vi "Build-raw-path.vi"(8 "error in (no error)":errorcluster, 11 "Reference in":T3) -> (0 "error out":errorcluster, 2 "Path":T1[](array[typedef]), 3 "Reference out":T3)   [LabVIEW 2013, in "HardwareCharacterization.lvlib" / "HC-ScanParser.lvclass"]
uses:
  HC-ScanParser.lvclass
  Object-reference.ctl
  Point-buffer.ctl
  SM1000-XML/Element-XML/Elements.ctl
  Path-buffer.ctl
  Property-buffer.ctl
  Units.ctl
  Speed.ctl
  HC-ScanParser.lvclass/HC-ScanParser.ctl
  SM1000-XML/Element-XML/Element-XML.lvclass
  Read Field properties.vi
  Read Laser properties.vi
  Read Elements.vi
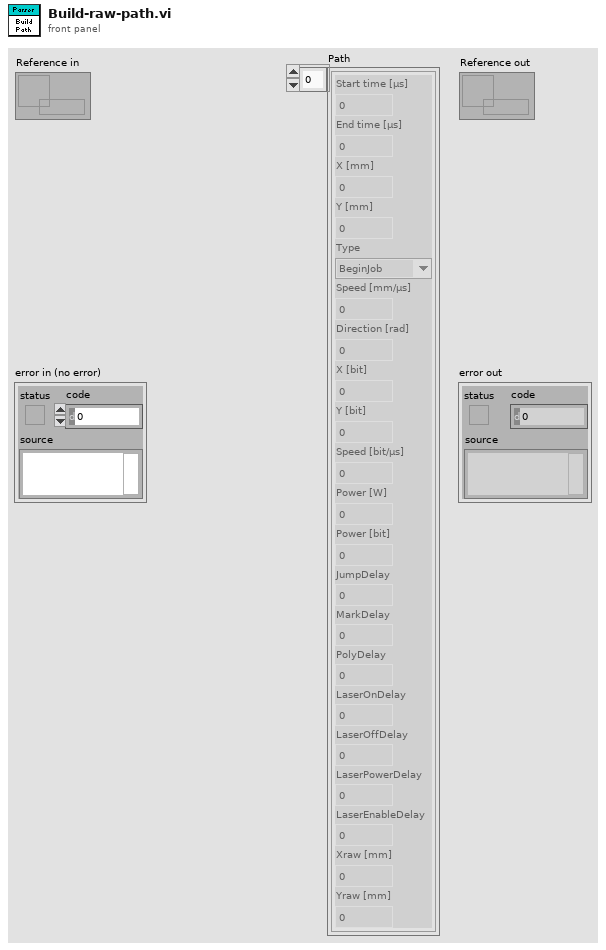
[diagram p1: front panel]
types:
  T1 = typedef "HardwareCharacterization.lvlib/HC-ScanParser.lvclass/Point-buffer.ctl" = cluster{"Start time [µs]":i64, "End time [µs]":i64, "X [mm]":dbl, "Y [mm]":dbl, "Type":T2, "Speed [mm/µs]":dbl, "Direction [rad]":dbl, "X [bit]":i16, "Y [bit]":i16, "Speed [bit/µs]":dbl, "Power [W]":dbl, "Power [bit]":u8, "JumpDelay":i64, "MarkDelay":i64, "PolyDelay":i64, "LaserOnDelay":i64, "LaserOffDelay":i64, "LaserPowerDelay":i64, "LaserEnableDelay":i64, "Xraw [mm]":dbl, "Yraw [mm]":dbl}
  T2 = typedef "HardwareCharacterization.lvlib/Element-XML.lvclass/Elements.ctl" = enum16{"BeginJob", "WriteDigital", "WriteAnalog", "Set", "ApplicationEvent", "JumpAbs", "MarkAbs", "JumpRel", "MarkRel", "LongDelay", "EndJob"}
  T3 = typedef "HardwareCharacterization.lvlib/HC-ScanParser.lvclass/Object-reference.ctl" = refnum<data-value>
  T4 = typedef "HardwareCharacterization.lvlib/HC-ScanParser.lvclass/Units.ctl" = enum16{"bits", "mm", "inch", "mils"}
  T5 = typedef "HardwareCharacterization.lvlib/HC-ScanParser.lvclass/Path-buffer.ctl" = cluster{"Previous point":T1, "Current point":T1, "Path":T1[], "Current properties":T6}
  T6 = typedef "HardwareCharacterization.lvlib/HC-ScanParser.lvclass/Property-buffer.ctl" = cluster{"ItemID":u32, "Start time":i64, "EffectiveOffset":dbl[], "EffectiveTranfsorm":dbl[][], "Z-Offset":sgl, "Units":T4, "LaserPower":u8, "Started":bool, "Enabled":bool, "FieldOffset":dbl[], "Offset":dbl[], "TransformEnable":bool, "XYCalFactor":dbl, "JumpSpeed":T7, "MarkSpeed":T7}
  T7 = typedef "HardwareCharacterization.lvlib/HC-ScanParser.lvclass/Speed.ctl" = cluster{"unit/us":dbl, "Tick interval us":u16, "Bits per interval":u16}
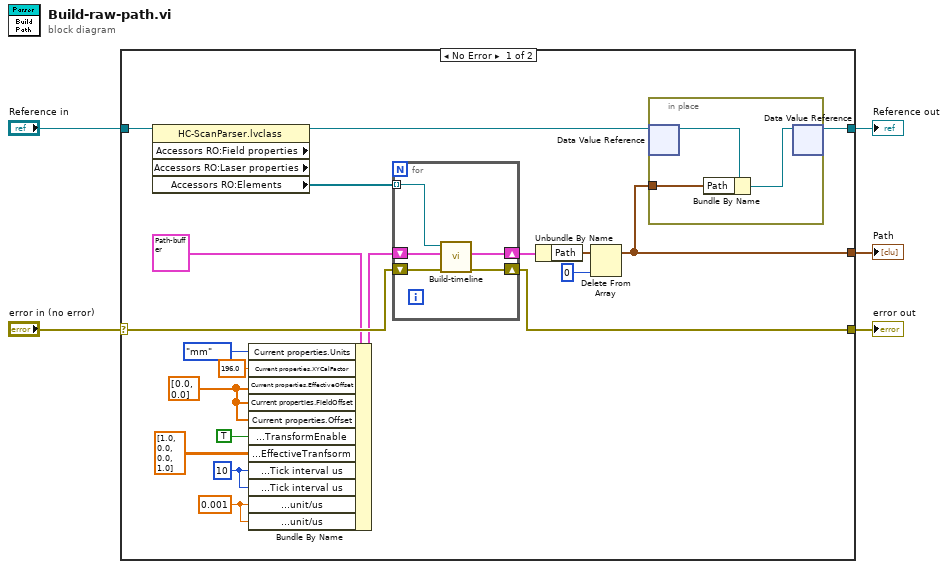
[diagram p0: block diagram]
diagram:
  n1 = case shown="No Error" "error in (no error)" {
    selector: "error in (no error)" -> [w20 w33]
    tunnel: [w19 w33] -> w4
    tunnel: [w21 w34] -> w2
    tunnel: "Reference in" -> [w24 w34]
    tunnel: [w6 _] -> w1
    frame No Error {
      w9 = 0.001 ("Current properties.JumpSpeed.unit/us")
      w10 = u16 10 ("Current properties.JumpSpeed.Tick interval us")
      w13 = dbl[] [0.0, 0.0] ("Current properties.EffectiveOffset")
      n2 = property class="HC-ScanParser.lvclass" props=["Accessors RO:Field properties", "Accessors RO:Laser properties", "Accessors RO:Elements"](reference=w24) -> (reference out=w22:T3, "Accessors RO:Elements"=w23:refnum<class "Element-XML.lvclass">[])  [unwired: 1 in, 3 out]
      n3 = Bundle By Name(cluster=T5 {"Previous point"={"Start time [µs]"=0, "End time [µs]"=0, "X [mm]"=0.0, "Y [mm]"=0.0, "Type"=enum."BeginJob", "Speed [mm/µs]"=0.0, "Direction [rad]"=0.0, "X [bit]"=0, "Y [bit]"=0, "Speed [bit/µs]"=0.0, "Power [W]"=0.0, "Power [bit]"=0, "JumpDelay"=0, "MarkDelay"=0, "PolyDelay"=0, "LaserOnDelay"=0, "LaserOffDelay"=0, "LaserPowerDelay"=0, "LaserEnableDelay"=0, "Xraw [mm]"=0.0, "Yraw [mm]"=0.0}, "Current point"={"Start time [µs]"=0, "End time [µs]"=0, "X [mm]"=0.0, "Y [mm]"=0.0, "Type"=enum."BeginJob", "Speed [mm/µs]"=0.0, "Direction [rad]"=0.0, "X [bit]"=0, "Y [bit]"=0, "Speed [bit/µs]"=0.0, "Power [W]"=0.0, "Power [bit]"=0, "JumpDelay"=0, "MarkDelay"=0, "PolyDelay"=0, "LaserOnDelay"=0, "LaserOffDelay"=0, "LaserPowerDelay"=0, "LaserEnableDelay"=0, "Xraw [mm]"=0.0, "Yraw [mm]"=0.0}, "Path"=[], "Current properties"={"ItemID"=0, "Start time"=0, "EffectiveOffset"=[], "EffectiveTranfsorm"=[], "Z-Offset"=0.0, "Units"=enum."bits", "LaserPower"=0, "Started"=FALSE, "Enabled"=FALSE, "FieldOffset"=[], "Offset"=[], "TransformEnable"=FALSE, "XYCalFactor"=0.0, "JumpSpeed"={"unit/us"=0.0, "Tick interval us"=0, "Bits per interval"=0}, "MarkSpeed"={"unit/us"=0.0, "Tick interval us"=0, "Bits per interval"=0}}} ("Path buffer"), "Current properties.Units"=Units."mm", "Current properties.XYCalFactor"=196.0, "Current properties.EffectiveOffset"=w13, "Current properties.FieldOffset"=w13, "Current properties.Offset"=w13, "Current properties.TransformEnable"=TRUE, "Current properties.EffectiveTranfsorm"=dbl[][] [[1.0, 0.0], [0.0, 1.0]] ("Current properties.EffectiveOffset"), "Current properties.JumpSpeed.Tick interval us"=w10, "Current properties.MarkSpeed.Tick interval us"=w10, "Current properties.JumpSpeed.unit/us"=w9, "Current properties.MarkSpeed.unit/us"=w9) -> (w16:T5)
      n4 = for {
        tunnel: w23 -> [w28] mode=indexing
        shift-right: [w30] -> w19
        shift-left: w20 -> [w31]
        shift-right: [w29] -> w18
        shift-left: w16 -> [w32]
        n5 = call-dynamic "Build-timeline.vi"("error in (no error)"=w31, "Temp-timeline in"=w32, "Element-XML in"=w28) -> ("error out"=w30:errorcluster, "Temp-timeline"=w29:T5)  [unwired: 6 in, 1 out]
      }
      n6 = Unbundle By Name(w18) -> ("Path"=w8:T1[])
      n7 = Delete From Array(array=w8, index=0) -> (array with subset deleted=w6:T1[])  [unwired: 1 in, 1 out]
      n8 = in-place {
        in-place-border: w6 -> [w25]
        n9 = in-place-dvr #1(w22) -> (w27:refnum<class "HC-ScanParser.lvclass">)  [unwired: 1 out]
        n10 = Bundle By Name(cluster=w27, "Path"=w25) -> (w26:refnum<class "HC-ScanParser.lvclass">)
        n11 = in-place-dvr #1(w26) -> (w21:T3)  [unwired: 1 out]
      }
    }
    frame Error {
    }
  }
  "error out" <- w4
  "Reference out" <- w2
  "Path" <- w1
